vi "2023 Read NavX.vi"() -> (0 "Heading":dbl, 1 "Pitch":dbl, 2 "Raw Values":T1 {"Accel X" format="%.8f"; "Accel Y" format="%.8f"; "Accel Z" format="%.8f"; "Gyro X" format="%.8f"; "Gyro Y" format="%.8f"; "Gyro Z" format="%.8f"; "Mag X" format="%.8f"; "Mag Y" format="%.8f"; "Mag Z" format="%.8f"}, 3 "Yaw":dbl, 4 "Roll":dbl)   [LabVIEW 2020]
uses:
  <vilib>/Rock Robotics/WPI/ThirdParty/Sensors/navX/_TypeDefs/FRIC_navX_DeviceNumbersTypeDef.ctl
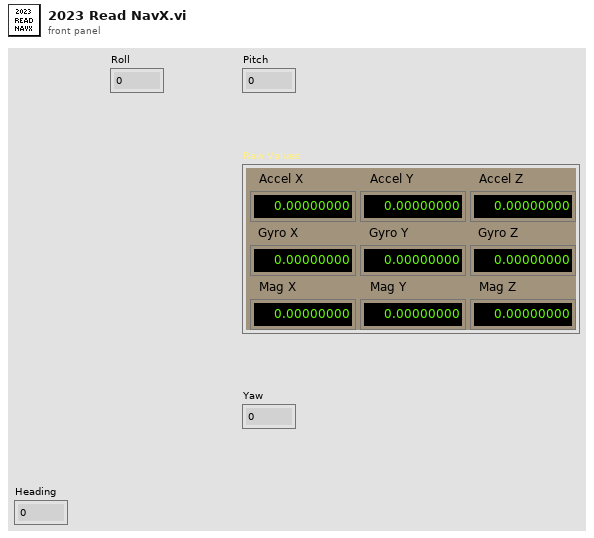
[diagram p1: front panel]
types:
  T1 = cluster{"Accel X":dbl, "Accel Y":dbl, "Accel Z":dbl, "Gyro X":dbl, "Gyro Y":dbl, "Gyro Z":dbl, "Mag X":dbl, "Mag Y":dbl, "Mag Z":dbl}
  T2 = typedef "FRIC_navX_DeviceNumbersTypeDef.ctl" = enum16{"Dev0", "Dev1", "Dev2", "Dev3"}
  T3 = cluster{"Yaw":dbl, "Roll":dbl, "Pitch":dbl, "Heading":dbl, "Fused Heading":dbl}
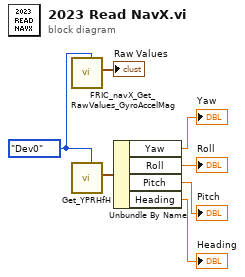
[diagram p0: block diagram]
diagram:
  w2 = FRIC_navX_DeviceNumbersTypeDef."Dev0" ("Device Number")
  n1 = call <vilib>:"FRIC_navX_Get_RawValues_GyroAccelMag.vi"("Device Number"=w2) -> ("Raw Values (out)"=→"Raw Values":T1)  [unwired: 10 in]
  n2 = call <vilib>:"Get_YPRHfH.vi"("Device Number"=w2) -> ("YRPHfH"=w3:T3)  [unwired: 10 in]
  n3 = Unbundle By Name(w3) -> ("Yaw"=→"Yaw":dbl, "Roll"=→"Roll":dbl, "Pitch"=→"Pitch":dbl, "Heading"=→"Heading":dbl)
